vi "fpga_Fund LP2 Process.vi"(0 "re":fxp<+/-,32,5>, 1 "reset":bool, 5 "im":fxp<+/-,32,5>, 7 "#Ch":fxp<+,5,5>=16.0, 9 "input valid":bool, 12 "ready for output":bool) -> (4 "re filtered":fxp<+/-,32,6> format="%.28g", 6 "im filtered":fxp<+/-,32,6> format="%.28g", 10 "output valid":bool, 14 "ready for input":bool)   [LabVIEW 2012, in "NI_EP_Protection_FPGA.lvlib"]
uses:
  <vilib>/addons/Electrical Power/Protection/NI_EP_Protection_FPGA.lvlib
  <vilib>/rvi/FXPMathLib/basic elements/FxpDiscreteDelay/XNode/nifxpmath_DiscreteDelay.xnode
  <vilib>/addons/Electrical Power/PQ/Resampling/NI_EP_Resample_FPGA.lvlib
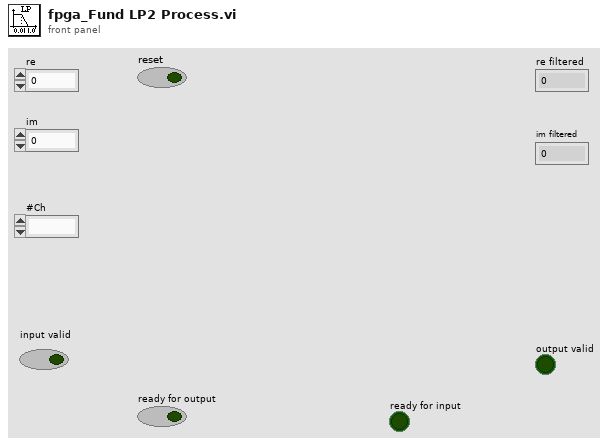
[diagram p1: front panel]
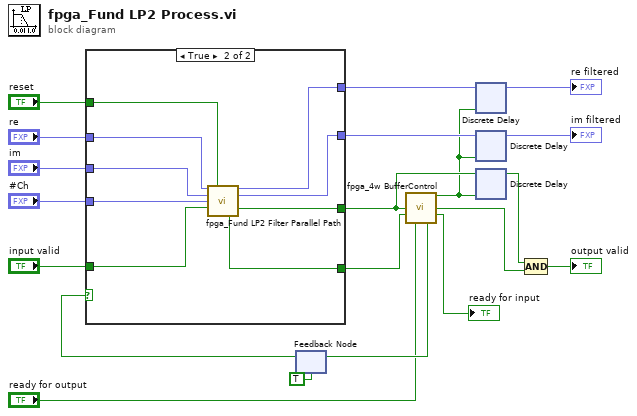
[diagram p0: block diagram]
diagram:
  n1 = feedback #1(TRUE ("logic enable")) -> (w15:bool)
  n2 = case shown="True" w15 {
    tunnel: "input valid" -> [_ w27]
    tunnel: "reset" -> [_ w25]
    tunnel: [_ w29] -> w8
    tunnel: [_ w28] -> w18
    tunnel: [_ w24] -> w4
    tunnel: [_ w23] -> w6
    tunnel: "re" -> [_ w22]
    tunnel: "#Ch" -> [_ w26]
    tunnel: "im" -> [_ w21]
    frame False {
    }
    frame True {
      n3 = call <vilib>:"fpga_Fund LP2 Filter Parallel Path.vi"("re"=w22, "reset"=w25, "im"=w21, "#Ch"=w26, "input valid"=w27) -> ("re filtered"=w24:fxp<+/-,32,6>, "im filtered"=w23:fxp<+/-,32,6>, "output valid"=w29:bool, "ready for input"=w28:bool)  [unwired: 7 in]
    }
  }
  n4 = call <vilib>:"fpga_4w BufferControl.vi"("DR"=w8, "RFI"=w18, "RFO"="ready for output") -> ("buff enable"=w3:bool, "output valid"=w17:bool, "ready for input"=→"ready for input":bool, "logic enable"=w16:bool)  [unwired: 9 in]
  n5 = feedback-in #1(w16) -> ()
  n6 = xnode "Discrete Delay"("D"=w4, "enable"=w3) -> ("Q"=→"re filtered":fxp<+/-,32,6>)
  n7 = xnode "Discrete Delay"("D"=w6, "enable"=w3) -> ("Q"=→"im filtered":fxp<+/-,32,6>)
  n8 = xnode "Discrete Delay"("D"=w8, "enable"=w3) -> ("Q"=w7:bool)
  n9 = Compound Arithmetic op=AND(w7, w17) -> (→"output valid":bool)
